vi "pm_load_nodes.vi"(8 "Error IN":errorcluster, 11 "HEKAdat.lvclass IN":refnum<class "HEKAdat.lvclass">) -> (0 "Error OUT":errorcluster, 3 "HEKAdat.lvclass OUT":refnum<class "HEKAdat.lvclass">)   [LabVIEW 2017, in "HEKAdat.lvclass"]
uses:
  HEKAdat.lvclass
  Tree.ctl
  HEKAdat.lvclass/HEKAdat.ctl
panel:
  in  "Tree":string(tree)
  out "Root":T1
  out "Node info":cluster{string, "Numeric":i32}[](array[cluster])
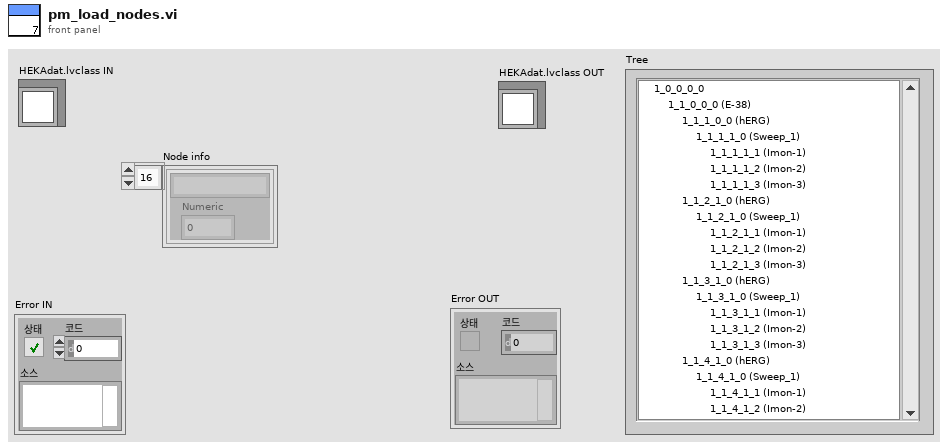
[diagram p1: front panel]
types:
  T1 = typedef "Tree.ctl" = cluster{"Label (Root)":string, "dataptr (Root)":u32, "nchildren (Root)":u32, "Group (1D)":cluster{"Label (Group)":string, "dataptr (Group)":u32, "nchildren (Group)":u32, "Series (1D)":cluster{"Label (Series)":string, "dataptr (Series)":u32, "nchildren (Series)":u32, "Sweep (1D)":cluster{"Label (Sweep)":string, "dataptr (Sweep)":u32, "nchildren (Sweep)":u32, "Trace (1D)":cluster{"dataptr (trace)":u32, "Label (Trace)":string, "Unit":string, "Unit_":dbl, "Xinterval":dbl, "nDatapoints":u32, "offset":u32, "Datascaler":dbl, "Trace":dbl[]}[]}[]}[]}[]}
  T2 = cluster{"Label (Group)":string, "dataptr (Group)":u32, "nchildren (Group)":u32, "Series (1D)":cluster{"Label (Series)":string, "dataptr (Series)":u32, "nchildren (Series)":u32, "Sweep (1D)":cluster{"Label (Sweep)":string, "dataptr (Sweep)":u32, "nchildren (Sweep)":u32, "Trace (1D)":cluster{"dataptr (trace)":u32, "Label (Trace)":string, "Unit":string, "Unit_":dbl, "Xinterval":dbl, "nDatapoints":u32, "offset":u32, "Datascaler":dbl, "Trace":dbl[]}[]}[]}[]}[]
  T3 = cluster{"Label (Group)":string, "dataptr (Group)":u32, "nchildren (Group)":u32, "Series (1D)":cluster{"Label (Series)":string, "dataptr (Series)":u32, "nchildren (Series)":u32, "Sweep (1D)":cluster{"Label (Sweep)":string, "dataptr (Sweep)":u32, "nchildren (Sweep)":u32, "Trace (1D)":cluster{"dataptr (trace)":u32, "Label (Trace)":string, "Unit":string, "Unit_":dbl, "Xinterval":dbl, "nDatapoints":u32, "offset":u32, "Datascaler":dbl, "Trace":dbl[]}[]}[]}[]}
  T4 = cluster{"Label (Series)":string, "dataptr (Series)":u32, "nchildren (Series)":u32, "Sweep (1D)":cluster{"Label (Sweep)":string, "dataptr (Sweep)":u32, "nchildren (Sweep)":u32, "Trace (1D)":cluster{"dataptr (trace)":u32, "Label (Trace)":string, "Unit":string, "Unit_":dbl, "Xinterval":dbl, "nDatapoints":u32, "offset":u32, "Datascaler":dbl, "Trace":dbl[]}[]}[]}[]
  T5 = cluster{"Label (Series)":string, "dataptr (Series)":u32, "nchildren (Series)":u32, "Sweep (1D)":cluster{"Label (Sweep)":string, "dataptr (Sweep)":u32, "nchildren (Sweep)":u32, "Trace (1D)":cluster{"dataptr (trace)":u32, "Label (Trace)":string, "Unit":string, "Unit_":dbl, "Xinterval":dbl, "nDatapoints":u32, "offset":u32, "Datascaler":dbl, "Trace":dbl[]}[]}[]}
  T6 = cluster{"Label (Sweep)":string, "dataptr (Sweep)":u32, "nchildren (Sweep)":u32, "Trace (1D)":cluster{"dataptr (trace)":u32, "Label (Trace)":string, "Unit":string, "Unit_":dbl, "Xinterval":dbl, "nDatapoints":u32, "offset":u32, "Datascaler":dbl, "Trace":dbl[]}[]}[]
  T7 = cluster{"Label (Sweep)":string, "dataptr (Sweep)":u32, "nchildren (Sweep)":u32, "Trace (1D)":cluster{"dataptr (trace)":u32, "Label (Trace)":string, "Unit":string, "Unit_":dbl, "Xinterval":dbl, "nDatapoints":u32, "offset":u32, "Datascaler":dbl, "Trace":dbl[]}[]}
  T8 = cluster{"dataptr (trace)":u32, "Label (Trace)":string, "Unit":string, "Unit_":dbl, "Xinterval":dbl, "nDatapoints":u32, "offset":u32, "Datascaler":dbl, "Trace":dbl[]}[]
  T9 = cluster{"dataptr (trace)":u32, "Label (Trace)":string, "Unit":string, "Unit_":dbl, "Xinterval":dbl, "nDatapoints":u32, "offset":u32, "Datascaler":dbl, "Trace":dbl[]}
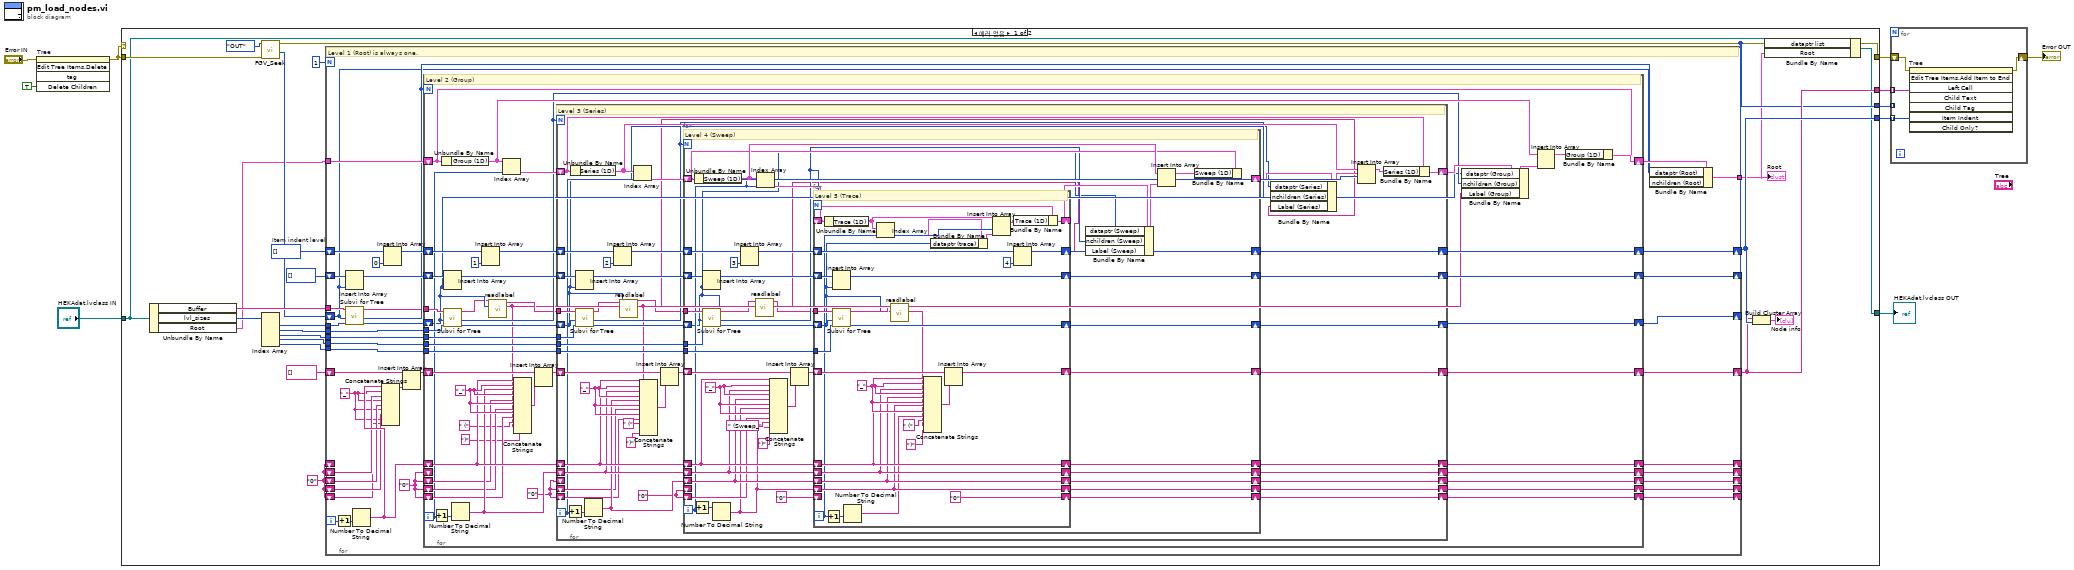
[diagram p0: block diagram]
diagram:
  n1 = invoke on="Tree" class="Tree (엄격한)" method="Edit Tree Items.Delete"(error in="Error IN", "Delete Children"=TRUE ("하위 아이템 삭제?")) -> (error out=w7:errorcluster)  [unwired: 3 in, 4 out]
  n2 = case shown="에러 없음" w7 {
    tunnel: w7 -> [w34 w241]
    tunnel: [w33 w241] -> w6
    tunnel: "HEKAdat.lvclass IN" -> [w16 w240]
    tunnel: [w14 w240] -> w9
    tunnel: [w18 _] -> w4
    tunnel: [w17 _] -> w3
    tunnel: [w15 _] -> w2
    frame No Error {
      w20 = "0"
      w22 = i32[] []  # Item indent level
      n3 = Unbundle By Name(w16) -> ("Buffer"=w25:string, "lvl_sizes"=w31:u32[], "Root"=w13:T1)
      n4 = call "FGV_Seek.vi"("Error IN"=w34, "IN or OUT"=enum16{"IN", "OUT"}."OUT") -> ("Error OUT"=w33:errorcluster, "Seek (con) OUT"=w21:u32)  [unwired: 8 in]
      n5 = Index Array(array=w31) -> (element #1=w26:u32, element #2=w30:u32, element #3=w29:u32, element #4=w28:u32, element #5=w27:u32)  [unwired: 5 in]
      n6 = for {
        N: 1 -> [_]
        tunnel: w30 -> [w73]
        tunnel: w29 -> [w72]
        tunnel: w28 -> [w71]
        tunnel: w27 -> [w70]
        tunnel: w26 -> [w69]
        tunnel: w25 -> [w67]
        shift-right: [w66] -> w15
        shift-left: u32[] [] -> [w65]
        shift-right: [w60] -> w18
        shift-left: w22 -> [w63]
        shift-right: [w59] -> _
        shift-left: w21 -> [w36]
        shift-right: [w58] -> _
        shift-left: w20 -> [_]
        shift-right: [w45] -> _
        shift-left: w20 -> [w50]
        shift-right: [w44] -> _
        shift-left: w20 -> [w49]
        shift-right: [w43] -> _
        shift-left: w20 -> [w48]
        shift-right: [w42] -> _
        shift-left: w20 -> [w46]
        shift-right: [w53] -> w17
        shift-left: string[] [] -> [w55]
        tunnel: w13 -> [w40]
        tunnel: [w37] -> w12
        i -> [w57]
        w41 = "0"
        w47 = "_" ("문자열")
        # "Level 1 (Root) is always one."
        n7 = Increment(x=w57) -> (x+1=w56:i32)
        n8 = Insert Into Array(array=w65, new element=w36) -> (w64:u32[])  [unwired: 1 in]
        n9 = call "Subvi for Tree.vi"("lvl size"=w69, "dataptr"=w36, "Buffer IN"=w67) -> ("dataptr for next lv"=w68:u32, "nchildren"=w38:u32, "Buffer OUT"=w35:string)  [unwired: 6 in]
        n10 = Number To Decimal String(number=w56) -> (decimal integer string=w51:string)  [unwired: 1 in]
        n11 = Concatenate Strings(w51, w47, w50, w47, w49, w47, w48, w47, w46) -> (w52:string)
        n12 = Insert Into Array(array=w63, new element=0 ("Numeric")) -> (w62:i32[])  [unwired: 1 in]
        n13 = Insert Into Array(array=w55, new element=w52) -> (w54:string[])  [unwired: 1 in]
        n14 = for {
          N: w38 -> [_]
          tunnel: w73 -> [w112]
          tunnel: w72 -> [w119]
          tunnel: w71 -> [w118]
          tunnel: w70 -> [w117]
          shift-right: [w116] -> w59
          shift-left: w68 -> [w79]
          shift-right: [w113] -> w66
          shift-left: w64 -> [w114]
          tunnel: w35 -> [w111]
          shift-right: [w106] -> w60
          shift-left: w62 -> [w109]
          shift-right: [w105] -> w58
          shift-left: w51 -> [w98]
          shift-right: [w93] -> w45
          shift-left: w41 -> [_]
          shift-right: [w92] -> w44
          shift-left: w41 -> [w96]
          shift-right: [w91] -> w43
          shift-left: w41 -> [w95]
          shift-right: [w90] -> w42
          shift-left: w41 -> [w94]
          shift-right: [w101] -> w53
          shift-left: w54 -> [w103]
          shift-right: [w84] -> w39
          shift-left: w40 -> [w83]
          i -> [w88]
          w89 = "0"
          w100 = "_" ("문자열")
          # "Level 2 (Group)"
          n15 = Increment(x=w88) -> (x+1=w104:i32)
          n16 = Unbundle By Name(w83) -> ("Group (1D)"=w87:T2)
          n17 = Insert Into Array(array=w114, new element=w79) -> (w115:u32[])  [unwired: 1 in]
          n18 = call "Subvi for Tree.vi"("lvl size"=w112, "dataptr"=w79, "Buffer IN"=w111) -> ("dataptr for next lv"=w110:u32, "nchildren"=w80:u32, "Buffer OUT"=w78:string)  [unwired: 6 in]
          n19 = Number To Decimal String(number=w104) -> (decimal integer string=w97:string)  [unwired: 1 in]
          n20 = Insert Into Array(array=w109, new element=1 ("Numeric")) -> (w108:i32[])  [unwired: 1 in]
          n21 = call "readlabel.vi"("ptr"=w79, "Buffer IN"=w78) -> ("Label"=w74:string, "Buffer OUT"=w77:string)  [unwired: 8 in]
          n22 = Index Array(array=w87, index=w88) -> (element=w85:T3)
          n23 = Concatenate Strings(w98, w100, w97, w100, w96, w100, w95, w100, w94, " (" ("문자열"), w74, ")" ("문자열")) -> (w99:string)
          n24 = Insert Into Array(array=w103, new element=w99) -> (w102:string[])  [unwired: 1 in]
          n25 = for {
            N: w80 -> [_]
            tunnel: w77 -> [w157]
            tunnel: w119 -> [w158]
            tunnel: w118 -> [w164]
            tunnel: w117 -> [w163]
            shift-right: [w160] -> w113
            shift-left: w115 -> [w161]
            shift-right: [w159] -> w116
            shift-left: w110 -> [w125]
            shift-right: [w153] -> w106
            shift-left: w108 -> [w156]
            shift-right: [w152] -> w105
            shift-left: w98 -> [w145]
            shift-right: [w140] -> w93
            shift-left: w97 -> [w144]
            shift-right: [w139] -> w92
            shift-left: w89 -> [_]
            shift-right: [w138] -> w91
            shift-left: w89 -> [w142]
            shift-right: [w137] -> w90
            shift-left: w89 -> [w141]
            shift-right: [w148] -> w101
            shift-left: w102 -> [w150]
            shift-right: [w130] -> w82
            shift-left: w85 -> [w129]
            i -> [w132]
            w136 = "0"
            w147 = "_" ("문자열")
            # "Level 3 (Series)"
            n26 = Increment(x=w132) -> (x+1=w151:i32)
            n27 = Unbundle By Name(w129) -> ("Series (1D)"=w133:T4)
            n28 = Insert Into Array(array=w161, new element=w125) -> (w162:u32[])  [unwired: 1 in]
            n29 = call "Subvi for Tree.vi"("lvl size"=w158, "dataptr"=w125, "Buffer IN"=w157) -> ("dataptr for next lv"=w135:u32, "nchildren"=w126:u32, "Buffer OUT"=w124:string)  [unwired: 6 in]
            n30 = Number To Decimal String(number=w151) -> (decimal integer string=w143:string)  [unwired: 1 in]
            n31 = Insert Into Array(array=w156, new element=2 ("Numeric")) -> (w154:i32[])  [unwired: 1 in]
            n32 = call "readlabel.vi"("ptr"=w125, "Buffer IN"=w124) -> ("Label"=w122:string, "Buffer OUT"=w123:string)  [unwired: 8 in]
            n33 = Index Array(array=w133, index=w132) -> (element=w134:T5)
            n34 = Concatenate Strings(w145, w147, w144, w147, w143, w147, w142, w147, w141, " (" ("문자열"), w122, ")" ("문자열")) -> (w146:string)
            n35 = Insert Into Array(array=w150, new element=w146) -> (w149:string[])  [unwired: 1 in]
            n36 = for {
              N: w126 -> [_]
              tunnel: w164 -> [w203]
              tunnel: w123 -> [w202]
              tunnel: w163 -> [w208]
              shift-right: [w207] -> w159
              shift-left: w135 -> [w170]
              shift-right: [w206] -> w160
              shift-left: w162 -> [w205]
              shift-right: [w198] -> w153
              shift-left: w154 -> [w200]
              shift-right: [w196] -> w152
              shift-left: w145 -> [w189]
              shift-right: [w186] -> w140
              shift-left: w144 -> [w188]
              shift-right: [w185] -> w139
              shift-left: w143 -> [w187]
              shift-right: [w184] -> w138
              shift-left: w136 -> [_]
              shift-right: [w183] -> w137
              shift-left: w136 -> [w182]
              shift-right: [w192] -> w148
              shift-left: w149 -> [w194]
              shift-right: [w175] -> w128
              shift-left: w134 -> [w176]
              i -> [w178]
              w191 = "_" ("문자열")
              # "Level 4 (Sweep)"
              n37 = Increment(x=w178) -> (x+1=w195:i32)
              n38 = Unbundle By Name(w176) -> ("Sweep (1D)"=w179:T6)
              n39 = Insert Into Array(array=w205, new element=w170) -> (w204:u32[])  [unwired: 1 in]
              n40 = call "Subvi for Tree.vi"("lvl size"=w203, "dataptr"=w170, "Buffer IN"=w202) -> ("dataptr for next lv"=w201:u32, "nchildren"=w172:u32, "Buffer OUT"=w171:string)  [unwired: 6 in]
              n41 = Number To Decimal String(number=w195) -> (decimal integer string=w166:string)  [unwired: 1 in]
              n42 = Insert Into Array(array=w200, new element=3 ("Numeric")) -> (w199:i32[])  [unwired: 1 in]
              n43 = call "readlabel.vi"("ptr"=w170, "Buffer IN"=w171) -> ("Label"=w168:string, "Buffer OUT"=w169:string)  [unwired: 8 in]
              n44 = Index Array(array=w179, index=w178) -> (element=w180:T7)
              n45 = Concatenate Strings(w189, w191, w188, w191, w187, w191, w166, w191, w182, " (Sweep_" ("문자열"), w166, ")" ("문자열")) -> (w190:string)
              n46 = Insert Into Array(array=w194, new element=w190) -> (w193:string[])  [unwired: 1 in]
              n47 = for {
                N: w172 -> [_]
                tunnel: w208 -> [w236]
                tunnel: w169 -> [w237]
                shift-right: [w235] -> w207
                shift-left: w201 -> [w212]
                shift-right: [w238] -> w206
                shift-left: w204 -> [w239]
                shift-right: [w232] -> w198
                shift-left: w199 -> [w234]
                shift-right: [w226] -> w196
                shift-left: w189 -> [w226]
                shift-right: [w225] -> w186
                shift-left: w188 -> [w225]
                shift-right: [w224] -> w185
                shift-left: w187 -> [w224]
                shift-right: [w223] -> w184
                shift-left: w166 -> [w223]
                shift-right: ["0"] -> w183
                shift-left: "0" -> [_]
                shift-right: [w229] -> w192
                shift-left: w193 -> [w230]
                shift-right: [w215] -> w174
                shift-left: w180 -> [w217]
                i -> [w218]
                w228 = "_" ("문자열")
                # "Level 5 (Trace)"
                n48 = Unbundle By Name(w217) -> ("Trace (1D)"=w220:T8)
                n49 = Increment(x=w218) -> (x+1=w231:i32)
                n50 = Insert Into Array(array=w239, new element=w212) -> (w238:u32[])  [unwired: 1 in]
                n51 = call "Subvi for Tree.vi"("lvl size"=w236, "dataptr"=w212, "Buffer IN"=w237) -> ("dataptr for next lv"=w235:u32, "Buffer OUT"=w213:string)  [unwired: 6 in, 1 out]
                n52 = Number To Decimal String(number=w231) -> (decimal integer string=w222:string)  [unwired: 1 in]
                n53 = Index Array(array=w220, index=w218) -> (element=w214:T9)
                n54 = call "readlabel.vi"("ptr"=w212, "Buffer IN"=w213) -> ("Label"=w209:string)  [unwired: 8 in, 1 out]
                n55 = Concatenate Strings(w226, w228, w225, w228, w224, w228, w223, w228, w222, " (" ("문자열"), w209, ")" ("문자열")) -> (w227:string)
                n56 = Bundle By Name(cluster=w214, "dataptr (trace)"=w212) -> (w219:T9)
                n57 = Insert Into Array(array=w230, new element=w227) -> (w229:string[])  [unwired: 1 in]
                n58 = Insert Into Array(array=w220, index=w218, new element=w219) -> (w216:T8)
                n59 = Bundle By Name(cluster=w217, "Trace (1D)"=w216) -> (w215:T7)
                n60 = Insert Into Array(array=w234, new element=4 ("Numeric")) -> (w232:i32[])  [unwired: 1 in]
              }
              n61 = Bundle By Name(cluster=w174, "dataptr (Sweep)"=w170, "nchildren (Sweep)"=w172, "Label (Sweep)"=w168) -> (w173:T7)
              n62 = Insert Into Array(array=w179, index=w178, new element=w173) -> (w177:T6)
              n63 = Bundle By Name(cluster=w176, "Sweep (1D)"=w177) -> (w175:T5)
            }
            n64 = Bundle By Name(cluster=w128, "dataptr (Series)"=w125, "nchildren (Series)"=w126, "Label (Series)"=w122) -> (w127:T5)
            n65 = Insert Into Array(array=w133, index=w132, new element=w127) -> (w131:T4)
            n66 = Bundle By Name(cluster=w129, "Series (1D)"=w131) -> (w130:T3)
          }
          n67 = Bundle By Name(cluster=w82, "dataptr (Group)"=w79, "nchildren (Group)"=w80, "Label (Group)"=w74) -> (w81:T3)
          n68 = Insert Into Array(array=w87, new element=w81) -> (w86:T2)  [unwired: 1 in]
          n69 = Bundle By Name(cluster=w83, "Group (1D)"=w86) -> (w84:T1)
        }
        n70 = Bundle By Name(cluster=w39, "dataptr (Root)"=w36, "nchildren (Root)"=w38) -> (w37:T1)
      }
      "Root" <- w12
      n71 = Build Cluster Array(w17, w18) -> (→"Node info":cluster{string, "Numeric":i32}[])
      n72 = Bundle By Name(cluster=w16, "dataptr list"=w15, "Root"=w12) -> (w14:refnum<class "HEKAdat.lvclass">)
    }
    frame Error {
    }
  }
  "HEKAdat.lvclass OUT" <- w9
  n73 = for {
    shift-right: [w244] -> w5
    shift-left: w6 -> [w245]
    tunnel: w4 -> [w243] mode=indexing
    tunnel: w3 -> [w242] mode=indexing
    tunnel: w2 -> [_] mode=indexing
    n74 = invoke on="Tree" class="Tree (엄격한)" method="Edit Tree Items.Add Item to End"(error in=w245, "Left Cell"=w242, "Item Indent"=w243) -> (error out=w244:errorcluster)  [unwired: 5 in, 7 out]
  }
  "Error OUT" <- w5
